vi "GetAxisData.vi"(0 "axis no":u8, 5 "device handle":i32, 11 "error in (no error)":T1) -> (2 "speed (°/s)":dbl, 3 "count":i32, 4 "moving":bool, 6 "StepWidth":i32, 8 "stop detected":bool, 10 "sensor error":bool, 12 "device handle 2":i32, 13 "position [µm/°/m°]":dbl, 14 "sensor disconnected":bool, 15 "error out":T1)   [LabVIEW 2019, in "Inst.Attocube-3DR.lvclass"]
uses:
  Inst.Attocube-3DR.lvclass
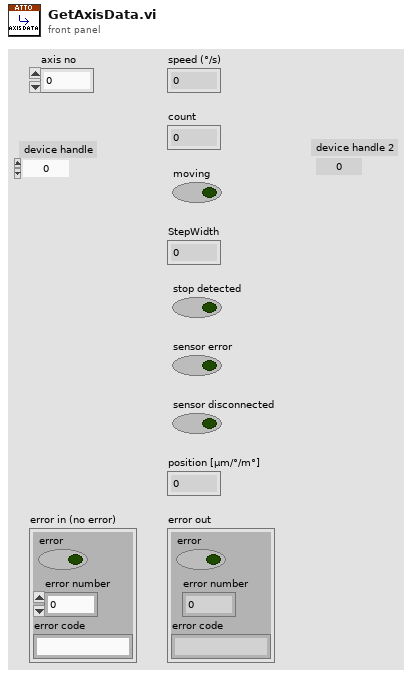
[diagram p1: front panel]
types:
  T1 = cluster{"error ":bool, "error number":i32, "error code":string}
  T2 = cluster{"moving":bool, "stop detected":bool, "sensor error":bool, "sensor disconnected":bool}
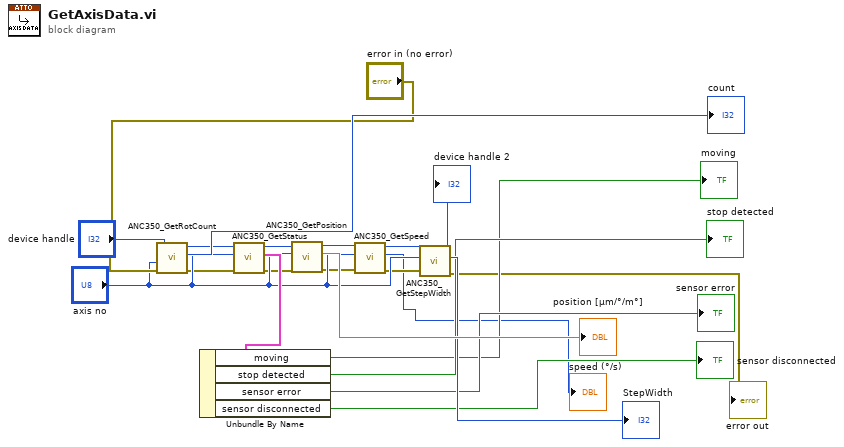
[diagram p0: block diagram]
diagram:
  n1 = call "ANC350_GetRotCount.vi"("error in"="error in (no error)", "axis no"="axis no", "device handle"="device handle") -> ("error out"=w9:T1, "count"=→"count":i32, "device handle"=w5:i32)  [unwired: 2 in]
  n2 = call "ANC350_GetStatus.vi"("error in"=w9, "axis no"="axis no", "device handle"=w5) -> ("error out"=w10:T1, "positioner status"=w14:T2, "device handle Out"=w6:i32)  [unwired: 1 in, 2 out]
  n3 = Unbundle By Name(w14) -> ("moving"=→"moving":bool, "stop detected"=→"stop detected":bool, "sensor error"=→"sensor error":bool, "sensor disconnected"=→"sensor disconnected":bool)
  n4 = call "ANC350_GetPosition.vi"("error in"=w10, "axis no"="axis no", "device handle"=w6) -> ("error out"=w11:T1, "position [µm/°/m°]"=→"position [µm/°/m°]":dbl, "device handle Out"=w7:i32)  [unwired: 2 in]
  n5 = call "ANC350_GetSpeed.vi"("error in"=w11, "axis no"="axis no", "device handle"=w7) -> ("error out"=w12:T1, "speed"=→"speed (°/s)":i32, "device handle"=w8:i32)  [unwired: 2 in]
  n6 = call "ANC350_GetStepWidth.vi"("error in"=w12, "axis no"="axis no", "device handle"=w8) -> ("error out"=→"error out":T1, "StepWidth"=→"StepWidth":i32, "device handle"=→"device handle 2":i32)  [unwired: 2 in]
